vi "Get for Constants Map.vi"(8 "error in (no error)":errorcluster, 11 "Constant Name":string) -> (0 "error out":errorcluster, 2 "Did it find it":bool, 3 "Value":dbl)   [LabVIEW 2013]
uses:
  Constants/Constants Global.vi
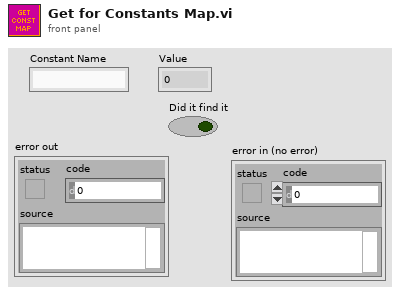
[diagram p1: front panel]
types:
  T1 = typedef "Constants Map typedef.ctl" = cluster{T2[]}[]
  T2 = typedef "Constants typedef V2.ctl" = cluster{"Constant Name":string, "Value":dbl}
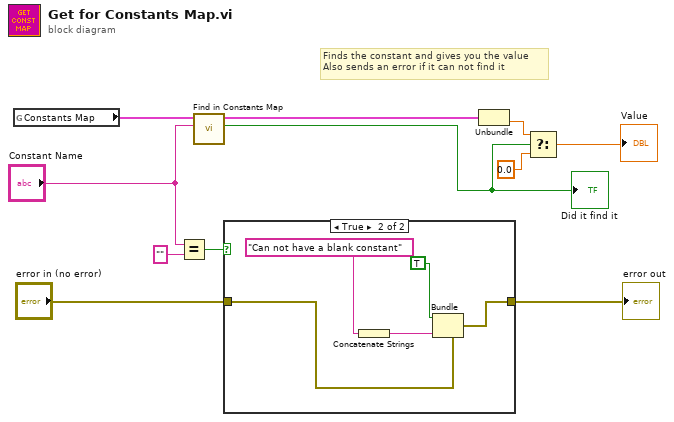
[diagram p0: block diagram]
diagram:
  # "Finds the constant and gives you the value\nAlso sends an error if it can not find it"
  n1 = global read "Constants Global.vi" "Constants Map"() -> (w11:T1)
  n2 = Equal?(x="Constant Name", y="") -> (x = y?=w7:bool)
  n3 = call "Find in Constants Map.vi"("Constant Name"="Constant Name", "Constants Map"=w11) -> ("Did it find it"=w2:bool, "Constants"=w10:T2)  [unwired: 6 in, 2 out]
  "Did it find it" <- w2
  n4 = case shown="True" w7 {
    tunnel: "error in (no error)" -> [w12 w17]
    tunnel: [w12 w16] -> w8
    frame False {
      # "No Error"
    }
    frame True {
      n5 = Concatenate Strings("Can not have a blank constant" ("string")) -> (w13:string)
      n6 = Bundle(cluster=w17, "status"=TRUE, "source"=w13) -> (w16:errorcluster)  [unwired: 1 in]
    }
  }
  "error out" <- w8
  n7 = Unbundle(w10) -> ("Value"=w4:dbl)  [unwired: 1 out]
  n8 = Select(t=w4, s=w2, f=0.0) -> (s? t:f=→"Value":dbl)
